vi "WebSocket Listen.vi"(4 "max payload bytes (5012)":i32=5012, 6 "WebSocket Connection Handler":refnum<class "WebSocket Connection Handler.lvclass">, 7 "net address":u32, 8 "log queue":refnum<queue>, 9 "quit?":refnum<notifier>, 10 "port":u16=8085, 11 "max connections (32)":u32=32) -> (0 "error out":errorcluster)   [LabVIEW 2019, in "WebSocket Server Toolkit.lvlib"]
doc: "<b>Description</b> Main entry point for the WebSocket server. This VI will continue to run until it receives a 'Quit' notification.\n\n<b>Inputs</b>\n<b>port</b>: Port to listen on.\n<b>net address</b>: Network address of the adapter to listen on. Defaults to all adapters.\n<b>log queue</b>: String-typed queue that will receive log notifications from the WebSocket server.\n<b>max connections</b>: The maximum number of concurrent connections to handle.\n<b>max payload bytes</b>: The maximum number of bytes to accept in a given payload.\n<b>WebSocket Connection Handler</b>: The connection handler that will accept WebSocket connections. You should implement a new connection handler and wire an object constant to this terminal.\n<b>quit?</b>: Boolean notifier. The webserver will quit if it receives a TRUE notification.\n\nBSD 3-Clause License\n\nCopyright (c) 2021, tauterra\nAll rights reserved.\n\nRedistribution and use in source and binary forms, with or without\nmodification, are permitted provided that the following conditions are met:\n\n1. Redistributions of source code must retain the above copyright notice, this\n list of conditions and the following disclaimer.\n\n2. Redistributions in binary form must reproduce the above copyright notice,\n this list of conditions and the following disclaimer in the documentation\n and/or other materials provided with the distribution.\n\n3. Neither the name of the copyright holder nor the names of its\n contributors may be used to endorse or promote products derived from\n this software without specific prior written permission.\n\nTHIS SOFTWARE IS PROVIDED BY THE COPYRIGHT HOLDERS AND CONTRIBUTORS \"AS IS\"\nAND ANY EXPRESS OR IMPLIED WARRANTIES, INCLUDING, BUT NOT LIMITED TO, THE\nIMPLIED WARRANTIES OF MERCHANTABILITY AND FITNESS FOR A PARTICULAR PURPOSE ARE\nDISCLAIMED. IN NO EVENT SHALL THE COPYRIGHT HOLDER OR CONTRIBUTORS BE LIABLE\nFOR ANY DIRECT, INDIRECT, INCIDENTAL, SPECIAL, EXEMPLARY, OR CONSEQUENTIAL\nDAMAGES (INCLUDING, BUT NOT LIMITED TO, PROCUREMENT OF SUBSTITUTE GOODS OR\nSERVICES; LOSS OF USE, DATA, OR PROFITS; OR BUSINESS INTERRUPTION) HOWEVER\nCAUSED AND ON ANY THEORY OF LIABILITY, WHETHER IN CONTRACT, STRICT LIABILITY,\nOR TORT (INCLUDING NEGLIGENCE OR OTHERWISE) ARISING IN ANY WAY OUT OF THE USE\nOF THIS SOFTWARE, EVEN IF ADVISED OF THE POSSIBILITY OF SUCH DAMAGE."
uses:
  WebSocket Server Toolkit.lvlib
  classes/WebSocket Connection Handler/WebSocket Connection Handler.lvclass
  7156248a-60e0-4153-86b0-aaecfde92c41.vi
  subVIs/handle_websocket_connection.vi
panel:
  out "# of connections":u32
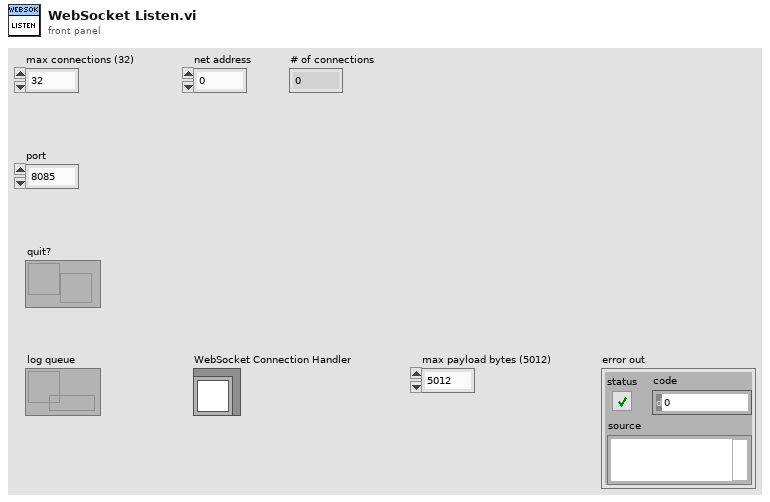
[diagram p1: front panel]
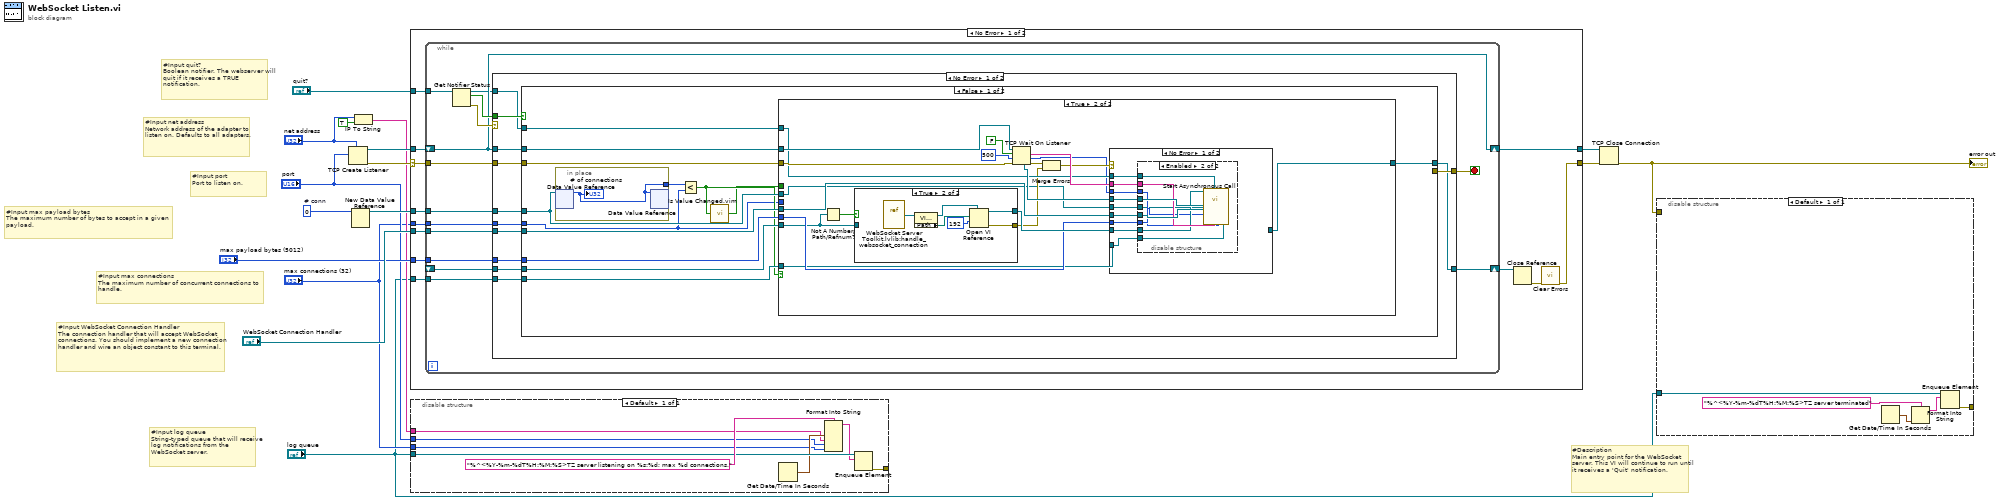
[diagram p0: block diagram]
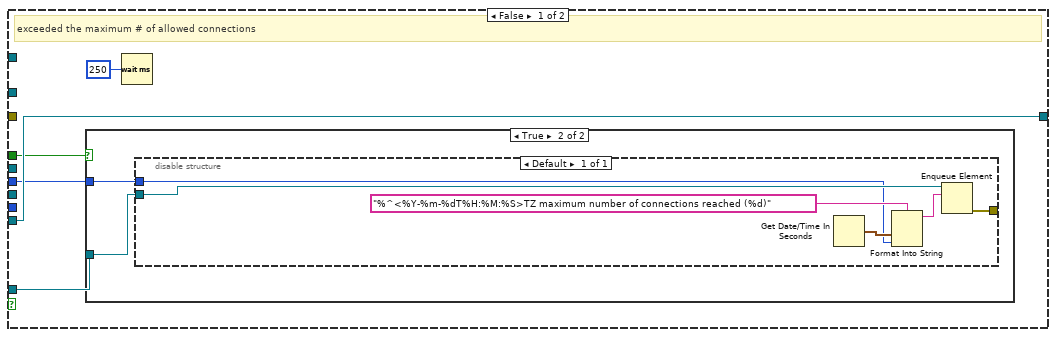
[diagram p2: hidden frame]
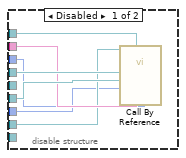
[diagram p5: hidden frame]
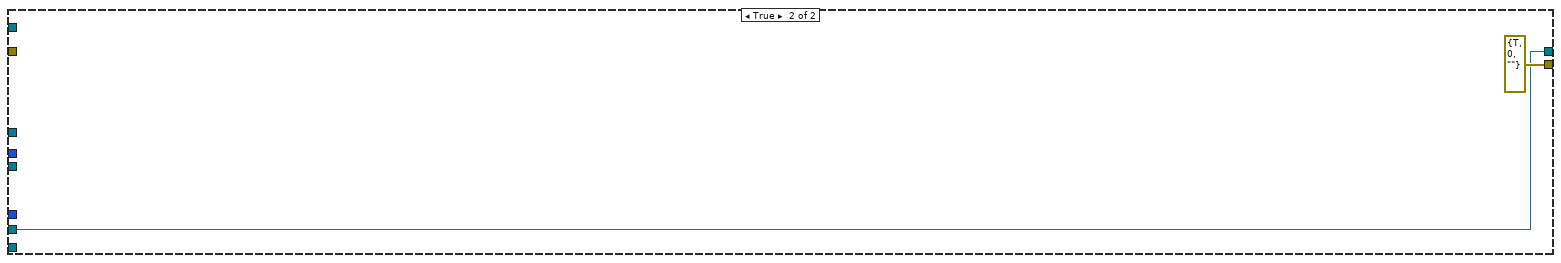
[diagram p7: hidden frame]
diagram:
  w9 = u32 0  # # conn
  # "#Input port\nPort to listen on."
  # "#Input net address\nNetwork address of the adapter to listen on. Defaults to all adapters."
  # "#Input log queue\nString-typed queue that will receive log notifications from the WebSocket server."
  # "#Input max connections\nThe maximum number of concurrent connections to handle."
  # "#Input max payload bytes\nThe maximum number of bytes to accept in a given payload."
  # "#Input WebSocket Connection Handler\nThe connection handler that will accept WebSocket connections. You should implement a new connection handler and wire an object constant to this terminal."
  # "#Input quit?\nBoolean notifier. The webserver will quit if it receives a TRUE notification."
  # "#Description\nMain entry point for the WebSocket server. This VI will continue to run until it receives a 'Quit' notification."
  n1 = TCP Create Listener(7:"net address", 10:"port") -> (0:w15:errorcluster, 3:w16:refnum<k5>)  [unwired: 3 in, 1 out]
  n2 = New Data Value Reference(data value=w9) -> (data value reference=w8:refnum<data-value>)  [unwired: 1 in, 1 out]
  n3 = IP To String(1:TRUE ("dot notation? (F)"), 2:"net address") -> (0:w6:string)
  n4 = case shown="No Error" w15 {
    selector: w15 -> [w27 w138]
    tunnel: w16 -> [w28 w139]
    tunnel: [w26 w139] -> w14
    tunnel: [w18 w138] -> w13
    tunnel: "WebSocket Connection Handler" -> [w25 _]
    tunnel: "quit?" -> [w24 _]
    tunnel: "max payload bytes (5012)" -> [w23 _]
    tunnel: w8 -> [w21 _]
    tunnel: "max connections (32)" -> [w20 _]
    tunnel: "log queue" -> [w19 _]
    frame No Error {
      n5 = while {
        tunnel: w27 -> [w42]
        tunnel: w25 -> [w41]
        shift-right: [w36] -> w26
        shift-left: w28 -> [w36]
        tunnel: w24 -> [w40]
        tunnel: w23 -> [w34]
        shift-right: [w33] -> w22
        shift-left: _ -> [w32]
        tunnel: w21 -> [w31]
        tunnel: w20 -> [w30]
        tunnel: w19 -> [w29]
        stop <- w38 stop-if-true
        n6 = Get Notifier Status(notifier=w40) -> (notifier out=w35:refnum<notifier>, current notification=w37:bool, error out=w39:errorcluster)  [unwired: 1 in, 2 out]
        n7 = case shown="No Error" w39 {
          selector: w39 -> [_ w137]
          tunnel: w36 -> [w54 _]
          tunnel: w42 -> [w53 _]
          tunnel: w41 -> [w52 _]
          tunnel: [w50 w137] -> w38
          tunnel: w37 -> [w51 _]
          tunnel: w35 -> [w49 _]
          tunnel: w34 -> [w48 _]
          tunnel: [w47 w136] -> w33
          tunnel: w32 -> [w46 w136]
          tunnel: w31 -> [w45 _]
          tunnel: w30 -> [w44 _]
          tunnel: w29 -> [w43 _]
          frame No Error {
            n8 = case shown="False" w51 {
              tunnel: w54 -> [w67 _]
              tunnel: w53 -> [w66 _]
              tunnel: w52 -> [w65 _]
              tunnel: [_ errorcluster {"status"=TRUE, "code"=0, "source"=""} ("error constant")] -> w50
              tunnel: w49 -> [w64 _]
              tunnel: w48 -> [w63 _]
              tunnel: [w62 w134] -> w47
              tunnel: w46 -> [w61 w134]
              tunnel: w45 -> [w60 _]
              tunnel: w44 -> [w55 _]
              tunnel: w43 -> [w58 _]
              frame False {
                n9 = in-place {
                  in-place-border: [w68] -> w59
                  n10 = in-place-dvr #1(w60) -> (w68:u32)  [unwired: 1 out]
                  "# of connections" <- w68
                  n11 = in-place-dvr #1(w68) -> ()  [unwired: 2 out]
                }
                n12 = Less?(x=w59, y=w55) -> (x < y?=w57:bool)
                n13 = call "Is Value Changed.vim"("value"=w57) -> ("changed or first call?"=w56:bool)
                n14 = case shown="True" w57 {
                  tunnel: w67 -> [_ w100]
                  tunnel: w66 -> [_ w99]
                  tunnel: w65 -> [_ w97]
                  tunnel: w64 -> [_ w90]
                  tunnel: w63 -> [_ w89]
                  tunnel: [w73 w88] -> w62
                  tunnel: w61 -> [w73 w86]
                  tunnel: w60 -> [_ w83]
                  tunnel: w58 -> [w70 w82]
                  tunnel: w56 -> [w71 _]
                  tunnel: w55 -> [w69 _]
                  frame False {
                    # "exceeded the maximum # of allowed connections"
                    n15 = case shown="True" w71 {
                      tunnel: w70 -> [_ w75]
                      tunnel: w69 -> [_ w74]
                      frame False {
                      }
                      frame True {
                        n16 = disable-structure shown="Default" {
                          disable-tunnel: w75 -> [w80]
                          disable-tunnel: [w77] -> _
                          disable-tunnel: w74 -> [w76]
                          frame Enabled {
                            n17 = Get Date/Time In Seconds() -> (seconds since 1Jan1904=w78:timestamp)
                            n18 = Format Into String(format string="%^<%Y-%m-%dT%H:%M:%S>TZ maximum number of connections reached (%d)", w78, w76) -> (resulting string=w79:string)  [unwired: 2 in, 1 out]
                            n19 = Enqueue Element(queue=w80, element=w79) -> (error out=w77:errorcluster)  [unwired: 2 in, 2 out]
                          }
                        }
                      }
                    }
                    n20 = Wait (ms)(milliseconds to wait=u32 250) -> ()  [unwired: 1 out]
                  }
                  frame True {
                    n21 = Not A Number/Path/Refnum?(number/path/refnum=w86) -> (NaN/Path/Refnum?=w87:bool)
                    n22 = case shown="True" w87 {
                      tunnel: [w101 w102] -> w93
                      tunnel: [_ w103] -> w85
                      tunnel: w86 -> [w101 _]
                      frame False {
                      }
                      frame True {
                        n23 = vi-ref "WebSocket Server Toolkit.lvlib:handle_websocket_connection.vi"() -> (w107:refnum<vi>)
                        n24 = property class="VI (strict)"(reference=w107) -> (reference out=w104:refnum<vi>, "Path"=w106:path)  [unwired: 1 in, 1 out]
                        n25 = Open VI Reference(type specifier VI Refnum (for type only)=w104, vi path=w106, options=192) -> (vi reference=w102:refnum<vi>, error out=w103:errorcluster)  [unwired: 3 in]
                      }
                    }
                    n26 = TCP Wait On Listener(8:w99, 9:500 ("timeout ms (wait forever: -1)"), 10:FALSE ("resolve remote address (T)"), 11:w100) -> (0:w94:errorcluster, 1:w84:u16, 2:w95:string, 4:w98:refnum<k5>)  [unwired: 1 out]
                    n27 = Merge Errors(w94, w85) -> (w92:errorcluster)
                    n28 = case shown="No Error" w92 {
                      tunnel: w98 -> [w116 _]
                      tunnel: w97 -> [w115 _]
                      tunnel: w95 -> [w114 _]
                      tunnel: w84 -> [w110 _]
                      tunnel: w93 -> [w113 w133]
                      tunnel: w90 -> [w112 _]
                      tunnel: w89 -> [w111 _]
                      tunnel: [_ w133] -> w88
                      tunnel: w83 -> [w109 _]
                      tunnel: w82 -> [w108 _]
                      frame No Error {
                        n29 = disable-structure shown="Enabled" {
                          disable-tunnel: w116 -> [w123 w132]
                          disable-tunnel: w115 -> [w122 w131]
                          disable-tunnel: w114 -> [w121 w130]
                          disable-tunnel: w113 -> [w120 w129]
                          disable-tunnel: w112 -> [w119 w128]
                          disable-tunnel: w111 -> [w118 w127]
                          disable-tunnel: w110 -> [w117 w126]
                          disable-tunnel: w109 -> [_ w125]
                          disable-tunnel: w108 -> [_ w124]
                          frame Disabled {
                            n30 = call-by-ref "?"(reference=w120, "remote port"=w117, "remote address"=w121, "quit?"=w119, "max payload bytes (5012)"=w118, "WebSocket Connection Handler"=w122, "TCP Network Connection in"=w123) -> ()  [unwired: 6 in, 3 out]
                          }
                          frame Enabled {
                            n31 = call-by-ref "Start Asynchronous Call"(reference=w129, "log queue"=w124, "remote port"=w126, "# conn."=w125, "remote address"=w130, "quit?"=w128, "max payload bytes (5012)"=w127, "WebSocket Connection Handler"=w131, "TCP Network Connection in"=w132) -> ()  [unwired: 4 in, 3 out]
                          }
                        }
                      }
                      frame Error {
                      }
                    }
                  }
                }
              }
              frame True {
              }
            }
          }
          frame Error {
          }
        }
      }
      n32 = Close Reference(reference=w22) -> (error out=w17:errorcluster)  [unwired: 1 in]
      n33 = call <vilib>:"Clear Errors.vi"("error in (no error)"=w17) -> ("error out"=w18:errorcluster)  [unwired: 5 in, 1 out]
    }
    frame Error {
    }
  }
  n34 = disable-structure shown="Default" {
    disable-tunnel: "log queue" -> [w146]
    disable-tunnel: [w143] -> _
    disable-tunnel: w6 -> [w142]
    disable-tunnel: "port" -> [w141]
    disable-tunnel: "max connections (32)" -> [w140]
    frame Enabled {
      n35 = Get Date/Time In Seconds() -> (seconds since 1Jan1904=w144:timestamp)
      n36 = Format Into String(format string="%^<%Y-%m-%dT%H:%M:%S>TZ server listening on %s:%d; max %d connections.", w144, w142, w141, w140) -> (resulting string=w145:string)  [unwired: 2 in, 1 out]
      n37 = Enqueue Element(queue=w146, element=w145) -> (error out=w143:errorcluster)  [unwired: 2 in, 2 out]
    }
  }
  n38 = TCP Close Connection(connection ID=w14, error in (no error)=w13) -> (error out=w2:errorcluster)  [unwired: 1 in, 1 out]
  "error out" <- w2
  n39 = disable-structure shown="Default" {
    disable-tunnel: [w149] -> _
    disable-tunnel: "log queue" -> [w148]
    disable-tunnel: w2 -> [_]
    frame Enabled {
      n40 = Get Date/Time In Seconds() -> (seconds since 1Jan1904=w150:timestamp)
      n41 = Format Into String(format string="%^<%Y-%m-%dT%H:%M:%S>TZ server terminated", w150) -> (resulting string=w151:string)  [unwired: 2 in, 1 out]
      n42 = Enqueue Element(queue=w148, element=w151) -> (error out=w149:errorcluster)  [unwired: 2 in, 2 out]
    }
  }
